vi "Admin functions test.vi"() -> ()   [LabVIEW 2021]
uses:
  Ethernet/Config Types/CAN Settings.ctl
  Ethernet/Config Types/Ethernet Settings.ctl
  Ethernet/Config Types/General Settings.ctl
  Protocol.ctl
  Ethernet/Ethernet.lvclass
  Battery Simulator 1200 Driver.lvclass
panel:
  in  "CAN Settings":T1={"Box ID"=1, "Publish Period (ms)"=5}
  in  "General Settings":T2
  in  "Ethernet Settings":T4={"IP Address"="192.168.1.100", "TCP (Command) Port"=12345, "TCP (Command) Read Interval (ms)"=10, "UDP (Reporting) Port"=54321, "UDP (Reporting) Write Interval (ms)"=5}
  out "Version":string
  out "General Settings":T2
  out "Ethernet Settings":T4={"IP Address"="192.168.1.100", "TCP (Command) Port"=12345, "TCP (Command) Read Interval (ms)"=10, "UDP (Reporting) Port"=54321, "UDP (Reporting) Write Interval (ms)"=5}
  out "CAN Settings":T1
  in  "Box IP address":string
  in  "UDP port":u16
  in  "TCP port":u16
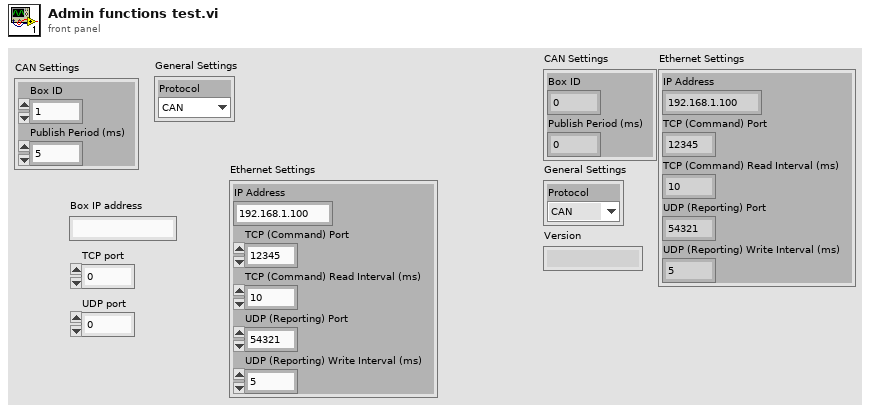
[diagram p1: front panel]
types:
  T1 = typedef "Battery Simulator 1200 LabVIEW Driver.lvlib/Ethernet.lvclass/CAN Settings.ctl" = cluster{"Box ID":i32, "Publish Period (ms)":i32}
  T2 = typedef "Battery Simulator 1200 LabVIEW Driver.lvlib/Ethernet.lvclass/General Settings.ctl" = cluster{"Protocol":T3}
  T3 = typedef "Battery Simulator 1200 LabVIEW Driver.lvlib/Battery Simulator 1200 Driver.lvclass/Protocol.ctl" = enum16{"CAN", "Ethernet"}
  T4 = typedef "Battery Simulator 1200 LabVIEW Driver.lvlib/Ethernet.lvclass/Ethernet Settings.ctl" = cluster{"IP Address":string, "TCP (Command) Port":u16, "TCP (Command) Read Interval (ms)":u32, "UDP (Reporting) Port":u16, "UDP (Reporting) Write Interval (ms)":u32}
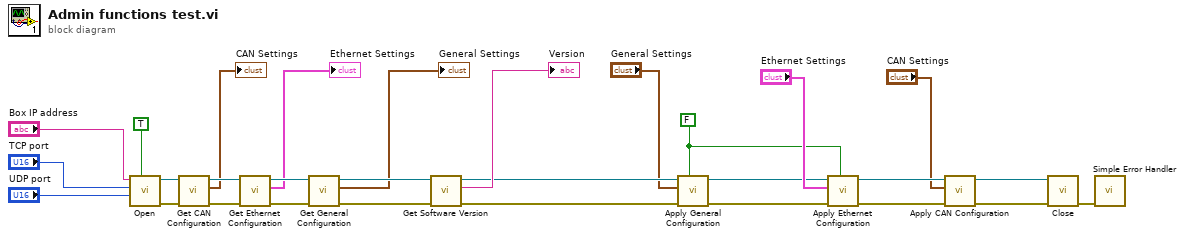
[diagram p0: block diagram]
diagram:
  w2 = FALSE ("Restart (T)")
  n1 = call "Open.vi"("Connect for Config Only? (F)"=TRUE ("Enable"), "UDP port"="UDP port", "TCP port"="TCP port", "Box IP address"="Box IP address") -> ("error out"=w17:errorcluster, "ENET out"=w21:refnum<class "Ethernet.lvclass">)  [unwired: 6 in]
  n2 = call "Get CAN Configuration.vi"("error in (no error)"=w17, "Ethernet in"=w21) -> ("error out"=w20:errorcluster, "CAN Settings"=→"CAN Settings":T1, "Ethernet out"=w24:refnum<class "Ethernet.lvclass">)  [unwired: 6 in, 1 out]
  n3 = call "Get Ethernet Configuration.vi"("error in (no error)"=w20, "Ethernet in"=w24) -> ("error out"=w19:errorcluster, "Ethernet Settings"=→"Ethernet Settings":T4, "Ethernet out"=w23:refnum<class "Ethernet.lvclass">)  [unwired: 6 in, 1 out]
  n4 = call "Get General Configuration.vi"("error in (no error)"=w19, "Ethernet in"=w23) -> ("error out"=w18:errorcluster, "General Settings"=→"General Settings":T2, "Ethernet out"=w22:refnum<class "Ethernet.lvclass">)  [unwired: 6 in, 1 out]
  n5 = call "Get Software Version.vi"("error in (no error)"=w18, "Ethernet in"=w22) -> ("error out"=w11:errorcluster, "Version"=→"Version":string, "Ethernet out"=w9:refnum<class "Ethernet.lvclass">)  [unwired: 7 in]
  n6 = call "Apply General Configuration.vi"("Restart (T)"=w2, "error in (no error)"=w11, "General Settings"="General Settings", "Ethernet in"=w9) -> ("error out"=w10:errorcluster, "Ethernet out"=w8:refnum<class "Ethernet.lvclass">)  [unwired: 6 in]
  n7 = call "Apply Ethernet Configuration.vi"("Restart (T)"=w2, "error in (no error)"=w10, "Ethernet Settings"="Ethernet Settings", "Ethernet in"=w8) -> ("error out"=w6:errorcluster, "Ethernet out"=w4:refnum<class "Ethernet.lvclass">)  [unwired: 6 in]
  n8 = call "Apply CAN Configuration.vi"("error in (no error)"=w6, "CAN Settings"="CAN Settings", "Ethernet in"=w4) -> ("error out"=w5:errorcluster, "Ethernet out"=w3:refnum<class "Ethernet.lvclass">)  [unwired: 7 in]
  n9 = call-dynamic "Close.vi"("error in (no error)"=w5, "ENET in"=w3) -> ("error out"=w29:errorcluster)  [unwired: 9 in]
  n10 = call <vilib>:"Simple Error Handler.vi"("error in (no error)"=w29) -> ()  [unwired: 4 in, 5 out]
